vi "MRC Configure Hardware.vi"(8 "error in (no error)":errorcluster, 11 "Hardware Resources in":T1={"MFC Definition"={"MFC Port"="", "MFC Enable"=TRUE, "Baud Rate"=0, "Interface type"=enum."RS-485", "Address"=0}, "Set Point Options"={"Setpoint Value"=0.0, "Mass Flow EU 2"="", "Setpoint Source"="", "Valve Mode"=""}, "Writer Queue"=refnum, "Enable"=FALSE, "Update Rate"=0, "MRC Chamber Enable"=FALSE, "Selected Gas"="", "Address String"=""} {"Set Point Options"."Setpoint Value" min=0.0 max=0.62495 format="%.5f"}) -> (0 "error out":errorcluster, 3 "Hardware Resources out":T1={"MFC Definition"={"MFC Port"="", "MFC Enable"=TRUE, "Baud Rate"=0, "Interface type"=enum."RS-485", "Address"=0}, "Set Point Options"={"Setpoint Value"=0.0, "Mass Flow EU 2"="", "Setpoint Source"="", "Valve Mode"=""}, "Writer Queue"=refnum, "Enable"=FALSE, "Update Rate"=0, "MRC Chamber Enable"=FALSE, "Selected Gas"="", "Address String"=""} {"Set Point Options"."Setpoint Value" min=0.0 max=0.62495 format="%.5f"})   [LabVIEW 2020, in "MRC Module.lvlib"]
doc: "Configure the hardware."
uses:
  MRC Module.lvlib
  MRC Configuration.ctl
  support/Message Queue/Message Cluster.ctl
  <vilib>/Instr/_visa.llb/VISA Configure Serial Port (Instr).vi
  support/Message Queue/Message Queue.lvlib
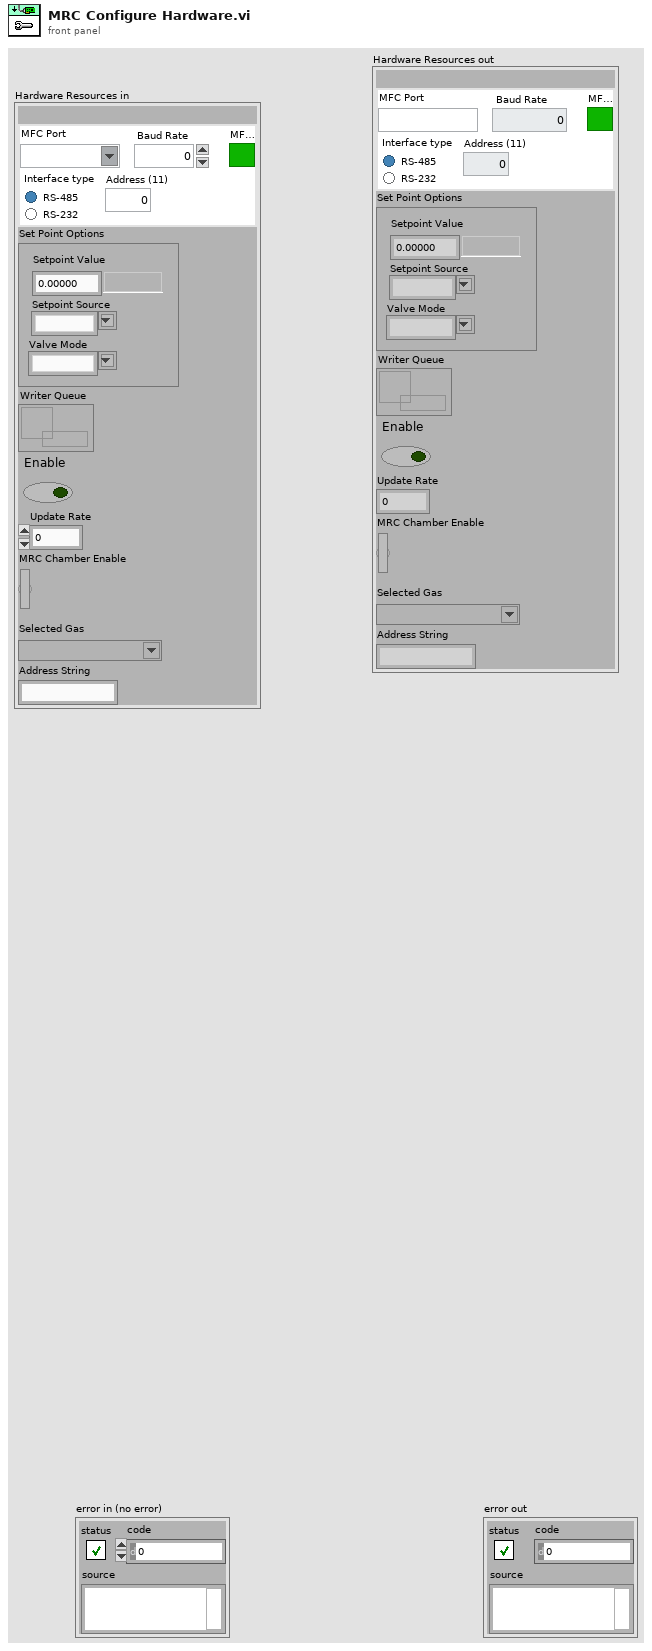
[diagram p1: front panel]
types:
  T1 = typedef "MRC Module.lvlib/MRC Configuration.ctl" = cluster{"MFC Definition":cluster{"MFC Port":refnum<visa-resource-name>, "MFC Enable":bool, "Baud Rate":i32, "Interface type":enum32{"RS-485", "RS-232"}, "Address":i32}, "Set Point Options":cluster{"Setpoint Value":dbl, "Mass Flow EU 2":string, "Setpoint Source":string, "Valve Mode":string}, "Writer Queue":refnum<queue>, "Enable":bool, "Update Rate":u32, "MRC Chamber Enable":bool, "Selected Gas":string, "Address String":string}
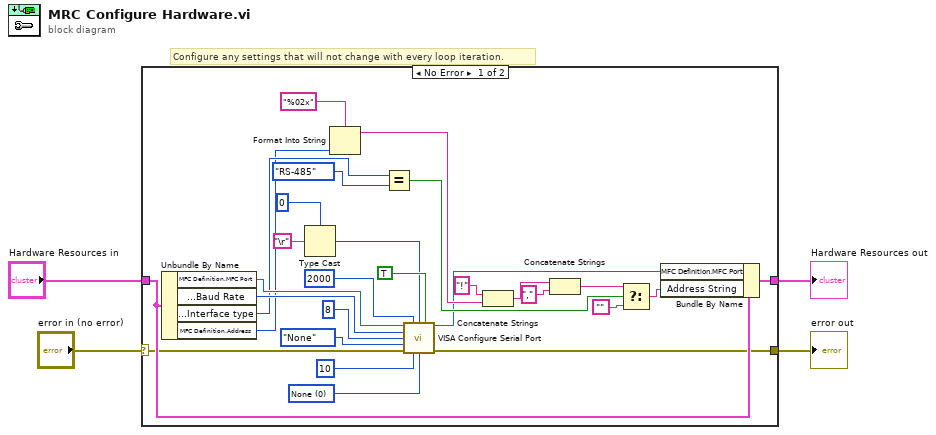
[diagram p0: block diagram]
diagram:
  # "Configure any settings that will not change with every loop iteration."
  n1 = case shown="No Error" "error in (no error)" {
    selector: "error in (no error)" -> [w5 w33]
    tunnel: [w6 w33] -> w3
    tunnel: "Hardware Resources in" -> [w31 w34]
    tunnel: [w32 w34] -> w1
    frame No Error {
      w10 = u16 0 items=["None", "XON/XOFF", "RTS/CTS", "XON/XOFF & RTS/CTS", "DTR/DSR", "XON/XOFF & DTR/DSR"] ("flow control (0:none)")
      n2 = Unbundle By Name(w31) -> ("MFC Definition.MFC Port"=w17:refnum<visa-resource-name>, "MFC Definition.Baud Rate"=w16:i32, "MFC Definition.Interface type"=w15:enum32{"RS-485", "RS-232"}, "MFC Definition.Address"=w12:i32)
      n3 = Type Cast(type=u8 0, x="\r") -> (*(type *) &x=w25:u8)
      n4 = Format Into String(format string="%02x", w12) -> (resulting string=w18:string)  [unwired: 2 in, 1 out]
      n5 = Equal?(x=w15, y=enum32{"RS-485", "RS-232"}."RS-485") -> (x = y?=w13:bool)
      n6 = call-poly "VISA Configure Serial Port"("VISA resource name"=w17, "timeout (10sec)"=2000, "termination char\n(0xA = '\\n' = LF)"=w25, "Enable Termination\nChar (T)"=TRUE, "baud rate (9600)"=w16, "data bits (8)"=8, "parity (0:none)"=enum16{"None", "Odd", "Even", "Mark", "Space"}."None", "error in (no error)"=w5, "stop bits (10: 1 bit)"=10, "flow control (0:none)"=w10) -> ("VISA resource name out"=w8:refnum<visa-resource-name>, "error out"=w6:errorcluster)  [unwired: 4 in]
      n7 = Concatenate Strings("!", w18) -> (w21:string)
      n8 = Concatenate Strings(w21, ",") -> (w20:string)
      n9 = Select(t=w20, s=w13, f="") -> (s? t:f=w7:string)
      n10 = Bundle By Name(cluster=w31, "MFC Definition.MFC Port"=w8, "Address String"=w7) -> (w32:T1)
    }
    frame Error {
    }
  }
  "Hardware Resources out" <- w1
  "error out" <- w3
